vi "MdsDescrText.vi"(0 "ValueIn":string) -> (1 "DescrId":i32, 2 "valueOut":string)   [LabVIEW 2011]
doc: "This VI will make a MDSplus descriptor from a 4-byte single 1D LabView array\n\nInputs:\n\n valueIn - single (required)\n\nOutputs:\n\n DescrId - int32 (recommended)\n valueOut - single (optional)"
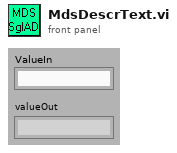
[diagram p1: front panel]
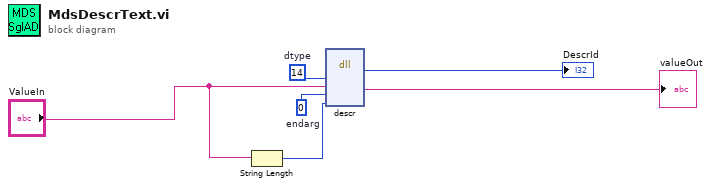
[diagram p0: block diagram]
diagram:
  w4 = 0  # endarg
  w6 = 14  # dtype
  n1 = String Length(string="ValueIn") -> (length=w1:i32)
  n2 = dll-call lib="MdsLib" fn="descr"("dtype"=w6, "value"="ValueIn", "endarg"=w4, "length"=w1) -> ("return type"=→"DescrId":i32, "value"=→"valueOut":string)  [unwired: 6 in, 2 out]
